vi "Lab16Sub.vi"(8 "error in (no error)":errorcluster, 9 "CI.Freq.Term":tag, 10 "Samples per \nMeasurement":i32=-1, 11 "Refnum in":refnum<k21>) -> (0 "error out":errorcluster, 2 "Measured Frequency":dbl format="%#_6p", 3 "Refnum out":refnum<k21>)   [LabVIEW 2022 SP3]
uses:
  <vilib>/DAQmx/configure/timing.llb/DAQmx Timing (Implicit).vi
  <vilib>/DAQmx/miscellaneous.llb/DAQmx Fill In Error Info.vi
  <vilib>/DAQmx/read.llb/DAQmx Read (Counter 1D DBL 1Chan NSamp).vi
  <resource>/objmgr/daqmx.rc
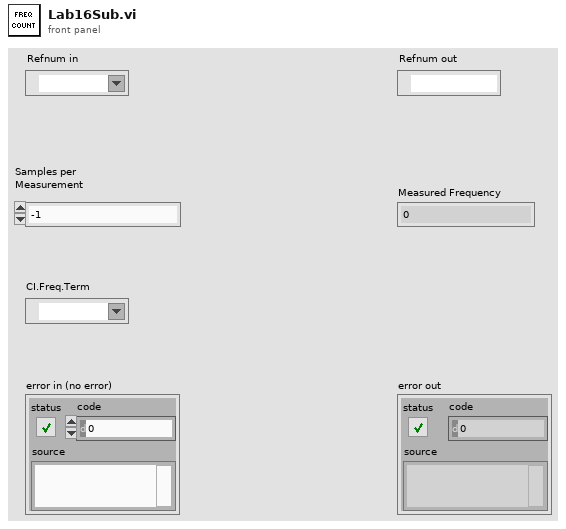
[diagram p1: front panel]
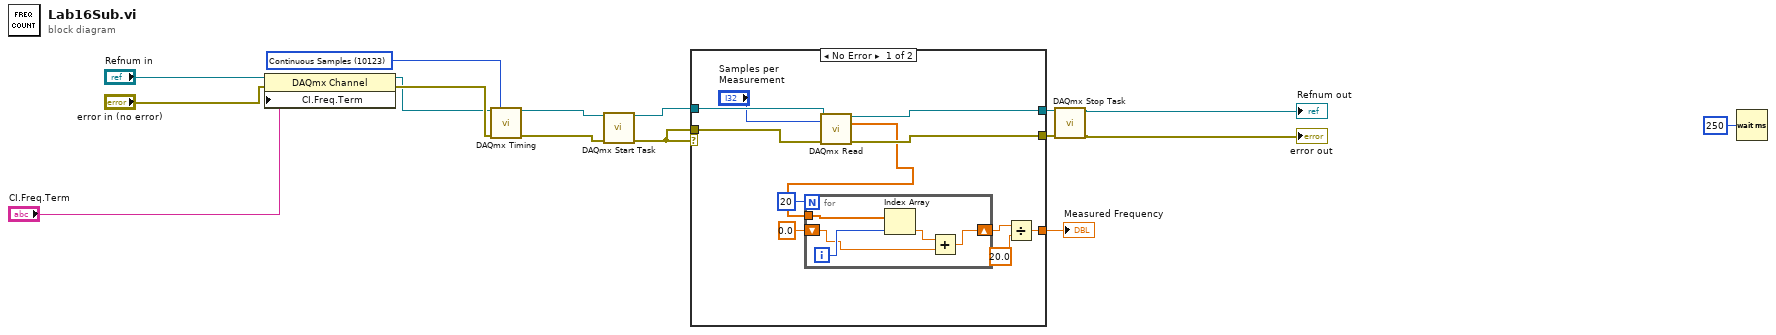
[diagram p0: block diagram]
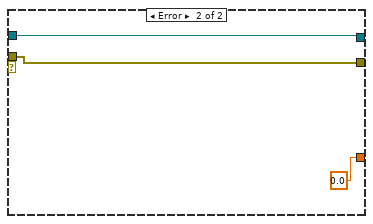
[diagram p2: hidden frame]
diagram:
  w16 = 10123 items=["Finite Samples"=10178, "Continuous Samples"=10123, "Hardware Timed Single Point"=12522] ("sample mode")
  n1 = property class="DAQmx Channel"(reference="Refnum in", error in="error in (no error)", "CI.Freq.Term"="CI.Freq.Term") -> (reference out=w14:refnum<k21>, error out=w15:errorcluster)
  n2 = call-poly <vilib>:"DAQmx Timing.vi"("task/channels in"=w14, "sample mode"=w16, "error in"=w15) -> ("task out"=w4:refnum<k21>, "error out"=w3:errorcluster)  [unwired: 11 in]
  n3 = call <vilib>:"DAQmx Start Task.vi"("task/channels in"=w4, "error in"=w3) -> ("task out"=w6:refnum<k21>, "error out"=w7:errorcluster)  [unwired: 12 in]
  n4 = case shown="No Error" w7 {
    tunnel: [w27 w35] -> w8
    tunnel: [w26 w34] -> w5
    tunnel: w7 -> [w25 w34]
    tunnel: w6 -> [w24 w35]
    tunnel: [w19 0.0] -> w10
    frame No Error {
      n5 = call-poly <vilib>:"DAQmx Read.vi"("task/channels in"=w24, "number of samples per channel"="Samples per \nMeasurement", "error in"=w25) -> ("task out"=w27:refnum<k21>, "data"=w22:dbl[], "error out"=w26:errorcluster)  [unwired: 10 in]
      n6 = for {
        N: 20 -> [_]
        tunnel: w22 -> [w32]
        shift-right: [w29] -> w17
        shift-left: 0.0 -> [w28]
        i -> [w31]
        n7 = Index Array(array=w32, index=w31) -> (element=w30:dbl)
        n8 = Add(x=w30, y=w28) -> (x+y=w29:dbl)
      }
      n9 = Divide(x=w17, y=20.0) -> (x/y=w19:dbl)
    }
    frame Error {
    }
  }
  "Measured Frequency" <- w10
  n10 = call <vilib>:"DAQmx Stop Task.vi"("task/channels in"=w8, "error in"=w5) -> ("task out"=→"Refnum out":refnum<k21>, "error out"=→"error out":errorcluster)  [unwired: 12 in]
  n11 = Wait (ms)(milliseconds to wait=u32 250) -> ()  [unwired: 1 out]
